vi "PhysicalChannel2Device.vi"() -> (2 "Associated Device":string[](array[string]), 3 "Physical Channels":tag[](array[tag]))   [LabVIEW 2013]
uses:
  <resource>/objmgr/daqmx.rc
panel:
  out "Devices":tag[](array[tag])
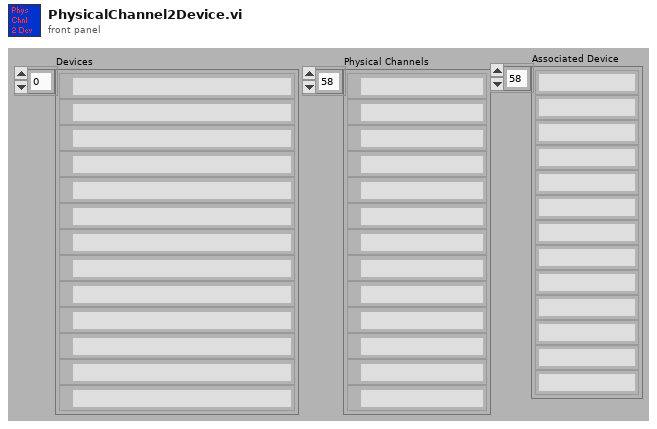
[diagram p1: front panel]
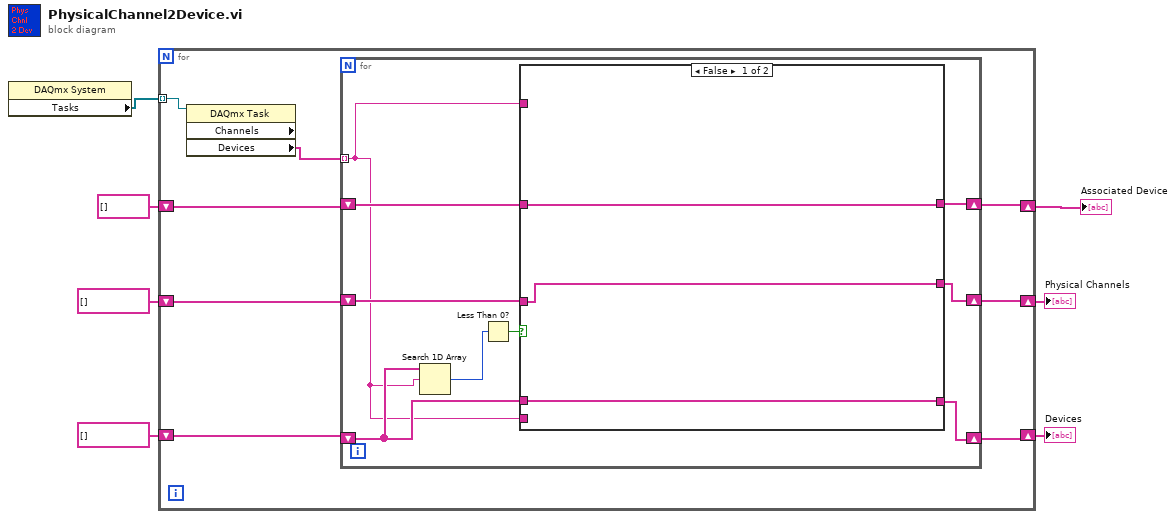
[diagram p0: block diagram]
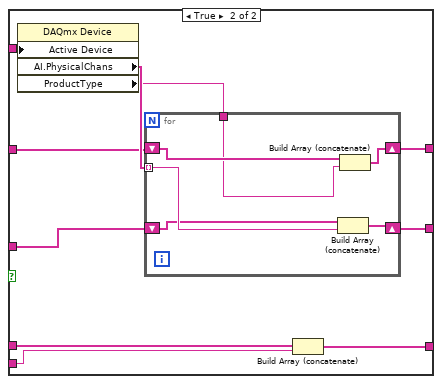
[diagram p2: hidden frame]
diagram:
  n1 = property class="DAQmx System"() -> ("Tasks"=w7:refnum<k21>[])  [unwired: 2 in, 2 out]
  n2 = for {
    tunnel: w7 -> [w15] mode=indexing
    shift-right: [w9] -> w2
    shift-left: string[] [] -> [w8]
    shift-right: [w13] -> w4
    shift-left: tag[] [] -> [w10]
    shift-right: [w12] -> w3
    shift-left: tag[] [] -> [w11]
    n3 = property class="DAQmx Task" props=["Channels", "Devices"](reference=w15) -> ("Devices"=w14:tag[])  [unwired: 1 in, 3 out]
    n4 = for {
      tunnel: w14 -> [w17] mode=indexing
      shift-right: [w24] -> w9
      shift-left: w8 -> [w23]
      shift-right: [w22] -> w13
      shift-left: w10 -> [w21]
      shift-right: [w16] -> w12
      shift-left: w11 -> [w18]
      n5 = Search 1D Array(1D array=w18, element=w17) -> (index of element=w19:i32)  [unwired: 1 out]
      n6 = Less Than 0?(x=w19) -> (x < 0?=w20:bool)
      n7 = case shown="False" w20 {
        tunnel: [w27 w36] -> w24
        tunnel: w23 -> [w27 w35]
        tunnel: w17 -> [_ w34]
        tunnel: [w26 w33] -> w22
        tunnel: w21 -> [w26 w32]
        tunnel: w18 -> [w25 w30]
        tunnel: w17 -> [_ w29]
        tunnel: [w25 w28] -> w16
        frame False {
        }
        frame True {
          n8 = property class="DAQmx Device"("Active Device"=w34) -> ("AI.PhysicalChans"=w37:tag[], "ProductType"=w31:string)  [unwired: 2 in, 2 out]
          n9 = for {
            shift-right: [w39] -> w36
            shift-left: w35 -> [w40]
            tunnel: w37 -> [w42] mode=indexing
            shift-right: [w43] -> w33
            shift-left: w32 -> [w41]
            tunnel: w31 -> [w38]
            n10 = Build Array (concatenate)(w41, w42) -> (w43:tag[])
            n11 = Build Array (concatenate)(w40, w38) -> (w39:string[])
          }
          n12 = Build Array (concatenate)(w30, w29) -> (w28:tag[])
        }
      }
    }
  }
  "Physical Channels" <- w4
  "Devices" <- w3
  "Associated Device" <- w2
